vi "ChannelsSetValues.vi"(8 "Timeout (ms)":i32, 9 "Values":dbl[](array[numeric]), 10 "Channel paths":string[](array[string]), 11 "Sequence Context In":refnum<k7>) -> (0 "error out":errorcluster, 1 "Channel Values Out":dbl[](array[numeric]), 2 "Channel paths out":string[](array[string]), 4 "Channel Units":string[](array[string]), 6 "timed out?":bool)   [LabVIEW 2015, in "ni-veristand-steps-runtime-lib.lvlib"]
uses:
  ni-veristand-steps-runtime-lib.lvlib
  <vilib>/NI Veristand/Execution/Workspace/NI VeriStand - Set Multiple Channel Values.vi
  <vilib>/NI Veristand/Execution/Workspace/NI VeriStand - Get Multiple Channel Values.vi
  <vilib>/NI Veristand/Execution/Workspace/NI_VS Workspace ExecutionAPI.lvlib
panel:
  out "Report":string
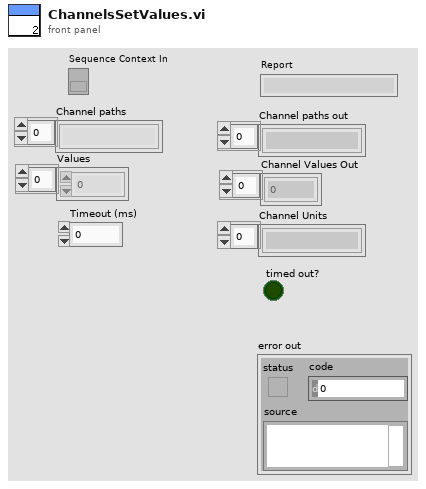
[diagram p1: front panel]
types:
  T1 = typedef "ni-veristand-steps-runtime-lib.lvlib/VeriStand dotNet References.ctl" = cluster{"Project Ref":refnum<k24>, "ModelManager":T2, "AlarmManager":T3, "ChannelFault":T4, "WorkspaceManager":T5}
  T2 = typedef "NI_VS ModelManager ExecutionAPI.lvlib/ModelManagerAPI.ctl" = refnum<k24>
  T3 = typedef "NI_VS AlarmManager ExecutionAPI.lvlib/AlarmManagerAPI.ctl" = refnum<k24>
  T4 = typedef "NI_VS ChannelFault ExecutionAPI.lvlib/ChannelFaultAPI.ctl" = refnum<k24>
  T5 = typedef "NI_VS Workspace ExecutionAPI.lvlib/WorkspaceAPI.ctl" = refnum<k24>
  T6 = typedef "NI_VS Workspace ExecutionAPI.lvlib/NodeInfo.ctl" = cluster{"Name":string, "FullPath":string, "Type":string, "IsChannel":bool, "Channel":cluster{"Unit":string, "Readable":bool, "Writable":bool, "Faultable":bool, "Scalable":bool, "RowDim":u32, "ColumnDim":u32, "Value Table Names":string[], "Value Table Values":dbl[]}, "IsWaveform":bool, "Waveform":cluster{"DataType":T7}}
  T7 = typedef "NI_VS Workspace ExecutionAPI.lvlib/Waveform Data Type.ctl" = enum16{"Double", "ComplexDouble"}
  T8 = typedef "TestStand - Status Monitor.ctl" = cluster{"Sequence Context":refnum<k7>, "Execution":refnum<k7>, "Termination Monitor":refnum<k7>}
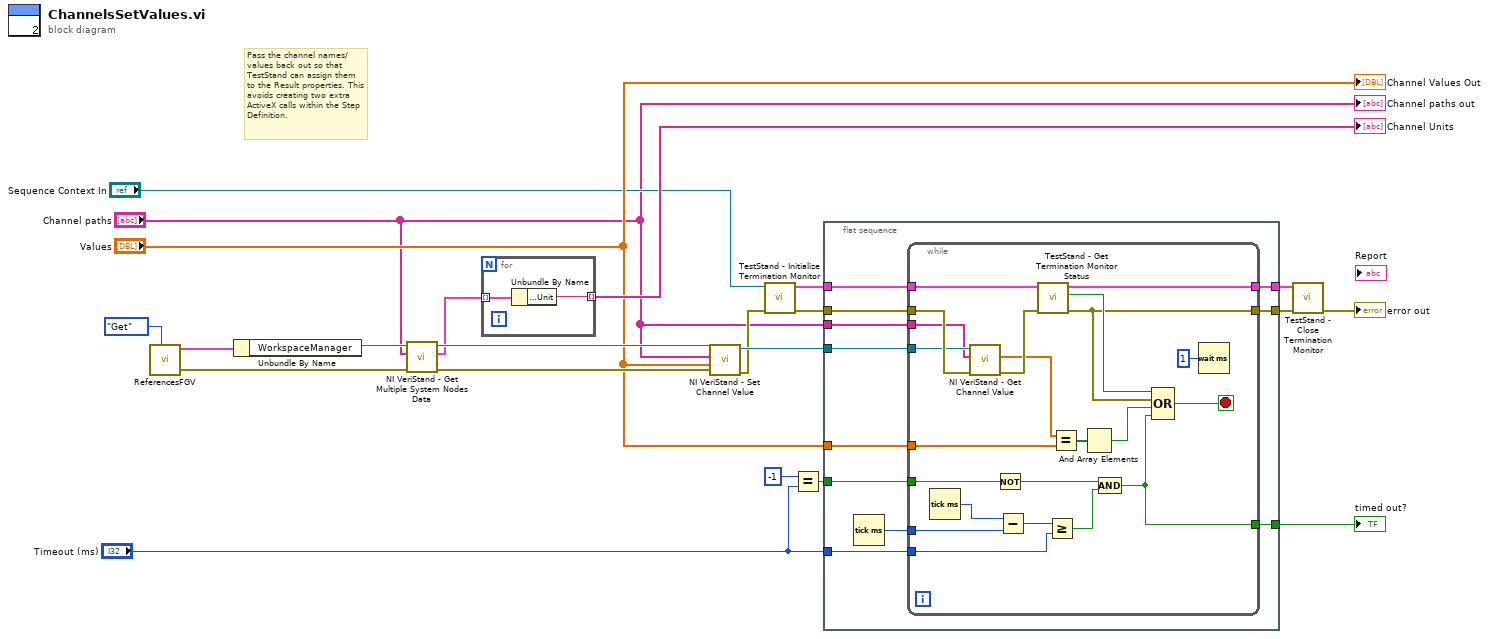
[diagram p0: block diagram]
diagram:
  # "Pass the channel names/values back out so that TestStand can assign them to the Result properties. This avoids creating two extra ActiveX calls within the Step Definition."
  n1 = call "ReferencesFGV.vi"("Get/Set"=enum16{"Get", "Set"}."Get") -> ("error out"=w8:errorcluster, "VeriStand dotNET Refs out"=w12:T1)  [unwired: 9 in]
  n2 = Unbundle By Name(w12) -> ("WorkspaceManager"=w9:T5)
  n3 = call <vilib>:"NI VeriStand - Get Multiple System Nodes Data.vi"("error in (no error)"=w8, "Node Paths"="Channel paths", "WorkspaceManager in"=w9) -> ("error out"=w6:errorcluster, "Nodes Data"=w5:T6[], "WorkspaceManager out"=w7:T5)  [unwired: 6 in]
  n4 = for {
    tunnel: w5 -> [w24] mode=indexing
    tunnel: [w23] -> w4 mode=indexing
    n5 = Unbundle By Name(w24) -> ("Channel.Unit"=w23:string)
  }
  "Channel Units" <- w4
  n6 = call-poly <vilib>:"NI VeriStand - Set Channel Value.vi"("error in (no error)"=w6, "Values"="Values", "Channels"="Channel paths", "WorkspaceManager in"=w7) -> ("error out"=w13:errorcluster, "WorkspaceManager out"=w18:T5)  [unwired: 6 in]
  n7 = call <vilib>:"TestStand - Initialize Termination Monitor.vi"("error in (no error)"=w13, "Sequence Context In"="Sequence Context In") -> ("error out"=w17:errorcluster, "Status Monitor Out"=w14:T8)  [unwired: 8 in]
  n8 = Equal?(x=-1, y="Timeout (ms)") -> (x = y?=w20:bool)
  n9 = flat-sequence {
    tunnel: w14 -> [w35]
    tunnel: [w34] -> w15
    tunnel: [w33] -> w16
    tunnel: w17 -> [w32]
    tunnel: w18 -> [w31]
    tunnel: w20 -> [w29]
    tunnel: [w28] -> w21
    tunnel: "Timeout (ms)" -> [w27]
    tunnel: "Channel paths" -> [w26]
    tunnel: "Values" -> [w25]
    frame #0 {
      n10 = Tick Count (ms)() -> (millisecond timer value=w30:u32)
      n11 = while {
        tunnel: w35 -> [w53]
        tunnel: [w52] -> w34
        tunnel: [w51] -> w33
        tunnel: w32 -> [w49]
        tunnel: w31 -> [w48]
        tunnel: w30 -> [w45]
        tunnel: w29 -> [w40]
        tunnel: [w41] -> w28
        tunnel: w27 -> [w38]
        tunnel: w26 -> [w37]
        tunnel: w25 -> [w36]
        stop <- w50 stop-if-true
        n12 = Tick Count (ms)() -> (millisecond timer value=w44:u32)
        n13 = call-poly <vilib>:"NI VeriStand - Get Channel Value.vi"("error in (no error)"=w49, "Channels"=w37, "WorkspaceManager in"=w48) -> ("error out"=w57:errorcluster, "Values"=w56:dbl[])  [unwired: 6 in, 1 out]
        n14 = Not(x=w40) -> (.not. x?=w39:bool)
        n15 = Subtract(x=w44, y=w45) -> (x-y=w43:u32)
        n16 = call <vilib>:"TestStand - Get Termination Monitor Status.vi"("error in (no error)"=w57, "Status Monitor In"=w53) -> ("error out"=w51:errorcluster, "Terminating or Aborting"=w55:bool, "Status Monitor Out"=w52:T8)  [unwired: 7 in]
        n17 = Greater Or Equal?(x=w43, y=w38) -> (x >= y?=w42:bool)
        n18 = Equal?(x=w56, y=w36) -> (x = y?=w47:bool[])
        n19 = And Array Elements(Boolean array=w47) -> (logical AND=w46:bool)
        n20 = Compound Arithmetic op=AND(w39, w42) -> (w41:bool)
        n21 = Compound Arithmetic op=OR(w55, w51, w46, w41) -> (w50:bool)
        n22 = Wait (ms)(milliseconds to wait=u32 1) -> ()  [unwired: 1 out]
      }
    }
  }
  n23 = call <vilib>:"TestStand - Close Termination Monitor.vi"("error in (no error)"=w16, "Status Monitor In"=w15) -> ("error out"=→"error out":errorcluster)  [unwired: 9 in]
  "Channel paths out" <- "Channel paths"
  "Channel Values Out" <- "Values"
  "timed out?" <- w21
